vi "Process.vi"(8 "error in (no error)":errorcluster, 11 "SMO.UI":refnum<class "SMO.UI.lvclass">) -> (0 "error out":errorcluster, 3 "SMO.UI out":refnum<class "SMO.UI.lvclass">)   [LabVIEW 2013, in "SMO.UI.lvclass"]
uses:
  SMO.UI.lvclass
  SMO/Typedefs/Parent Call--Enum.ctl
  SMO/SMO.lvclass
panel:
  in  "OK":bool
  out "Copyright":string="JKI State Machine Objects™\nhttp://jki.net/state-machine-objects/\nCopyright (C) 2005-2015, JKI <info@jki.net>\nALL RIGHTS RESERVED\n\nFor instructions on how to use the JKI State Machine Objects, examples and video tutorials, visit:\nhttp://jki.net/state-machine-objects/\n"
  # "JKI SMO UI"
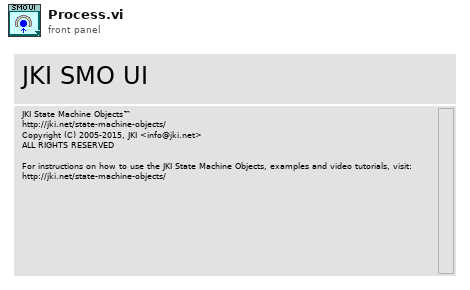
[diagram p1: front panel]
types:
  T1 = typedef "SMO.lvclass/Parent Call--Enum.ctl" = enum16{"Allows parent to run", "Does not request parent to run"}
  T2 = enum32{"invalid app kind", "Development System", "Run Time System", "Student Edition", "Embedded LabVIEW", "Evaluation", "Custom"}
  T3 = enum32{"Invalid", "Standard", "Closed", "Hidden", "Minimized", "Maximized"}
  T4 = cluster{"Core":cluster{"Current VI Reference":refnum<vi>, "Close Panel on Exit?":bool, "error":errorcluster}, "Self Ref":refnum<class "SMO.UI.lvclass">}
  T5 = cluster{"Current VI Reference":refnum<vi>, "Close Panel on Exit?":bool, "error":errorcluster}
  T6 = typedef "SMO.lvclass/Protected Events.ctl" = cluster{"StopProcesses":refnum<user-event>, "AbortProcesses":refnum<user-event>}
  T7 = typedef "SMO.UI.lvclass/PrivateEvents--Cluster.ctl" = cluster{"Show-Hide UI":refnum<user-event>}
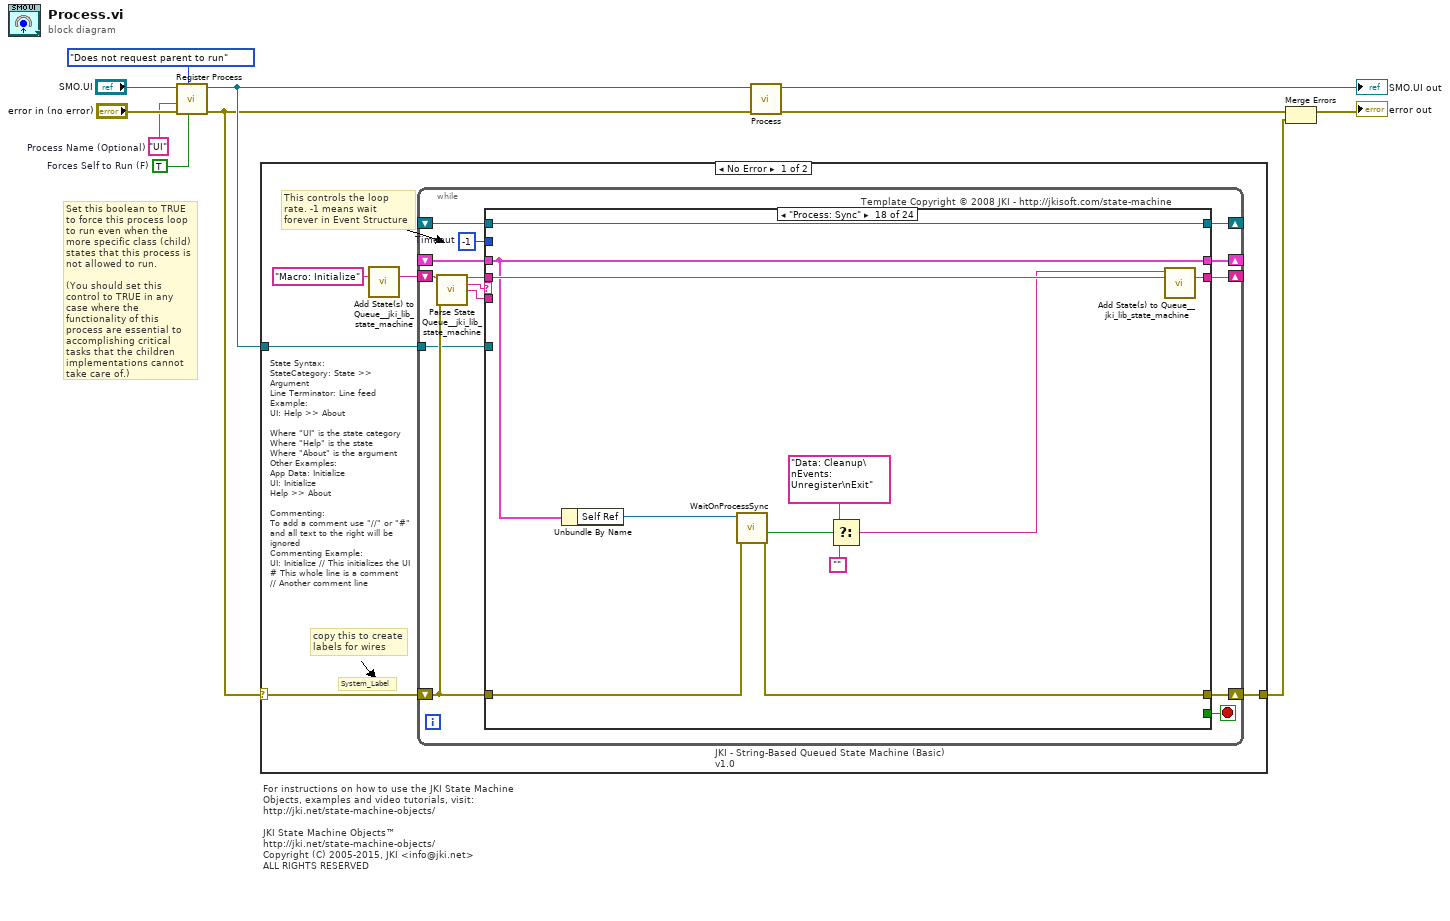
[diagram p0: block diagram]
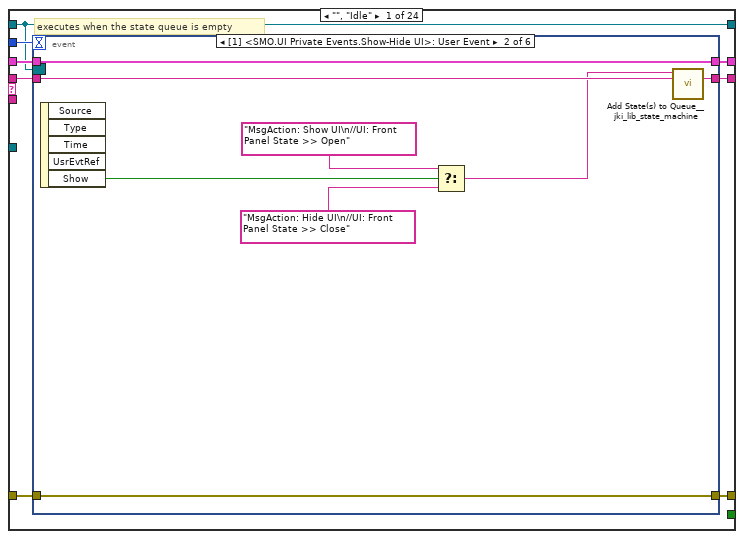
[diagram p2: hidden frame]
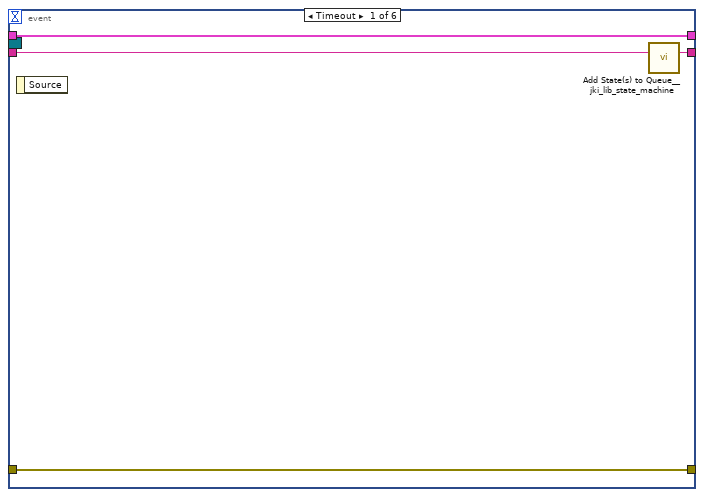
[diagram p3: hidden frame]
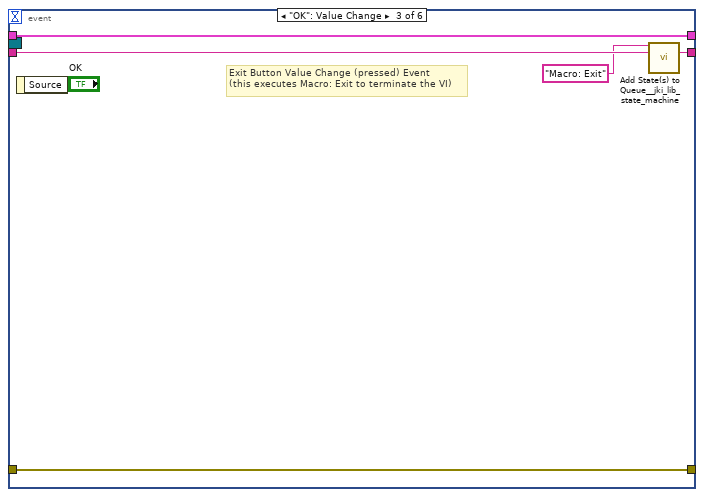
[diagram p4: hidden frame]
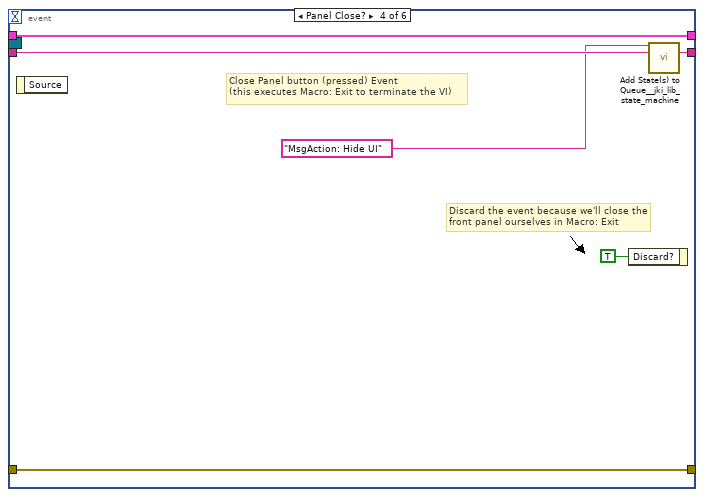
[diagram p5: hidden frame]
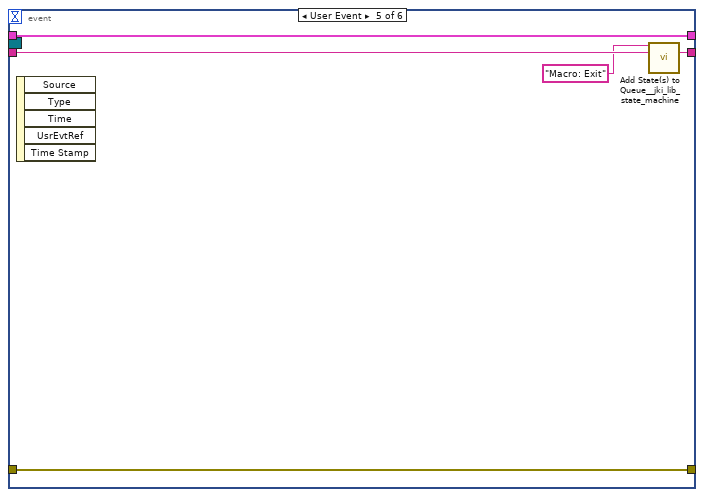
[diagram p6: hidden frame]
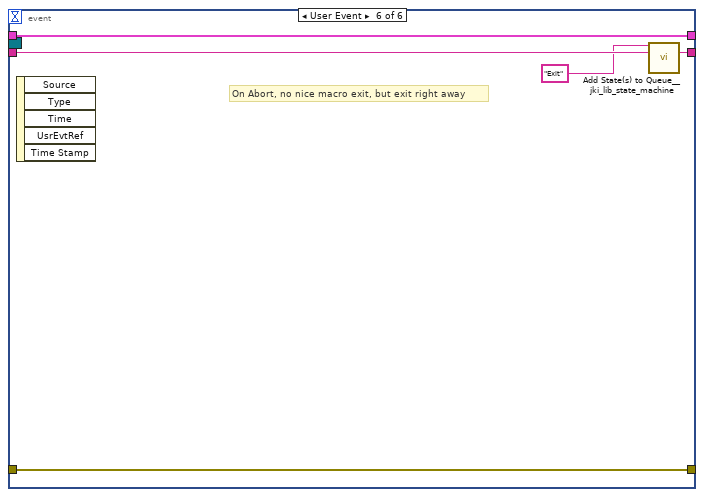
[diagram p7: hidden frame]
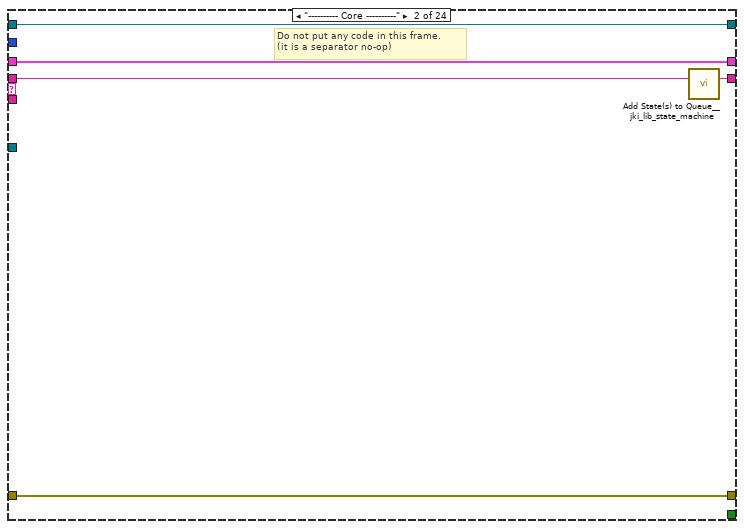
[diagram p8: hidden frame]
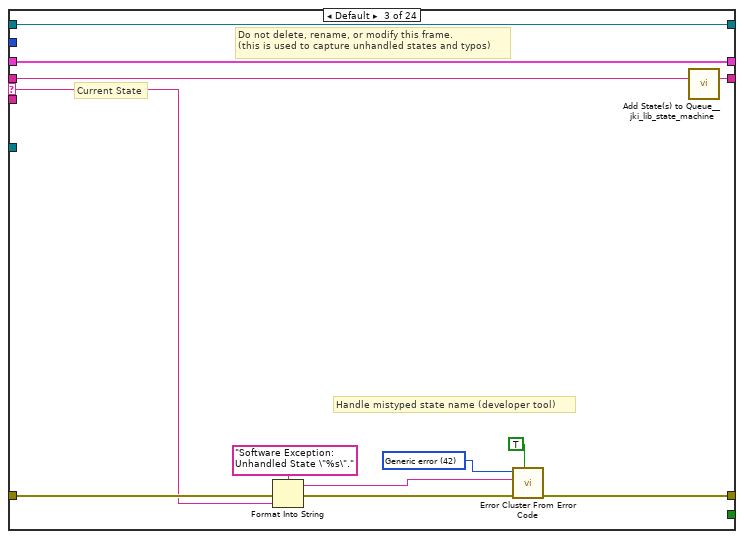
[diagram p9: hidden frame]
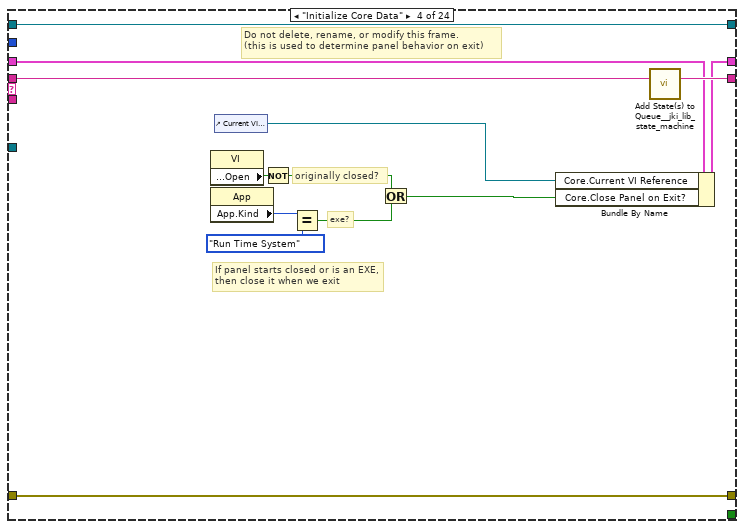
[diagram p10: hidden frame]
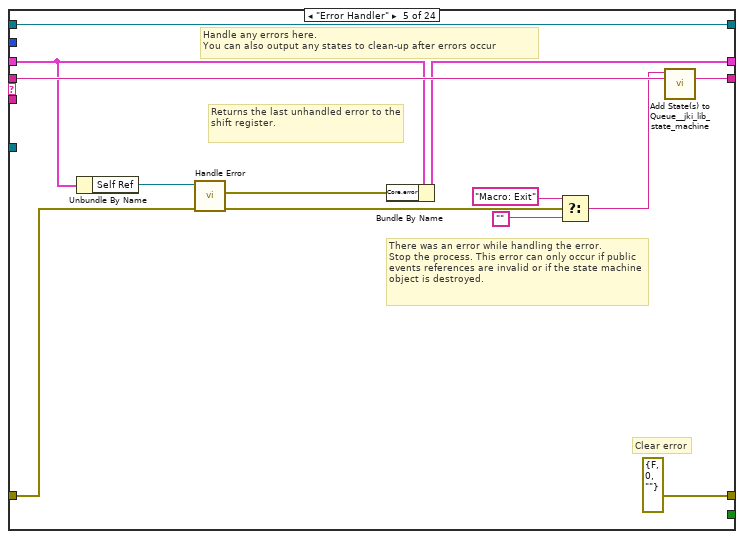
[diagram p11: hidden frame]
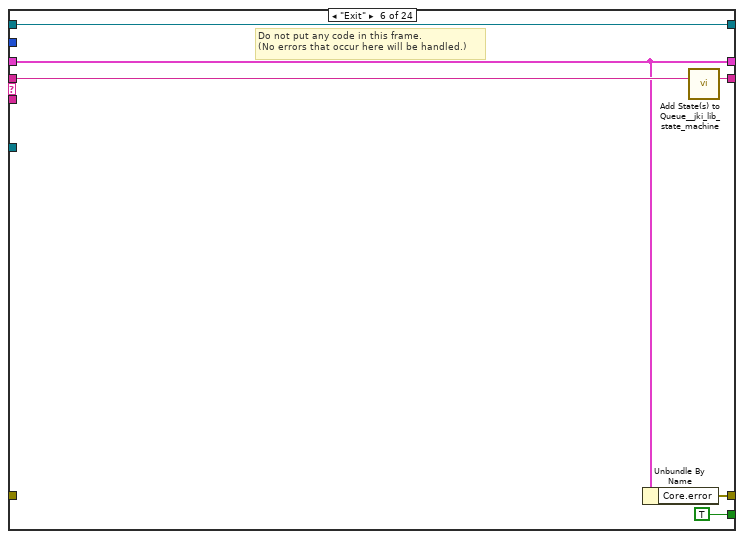
[diagram p12: hidden frame]
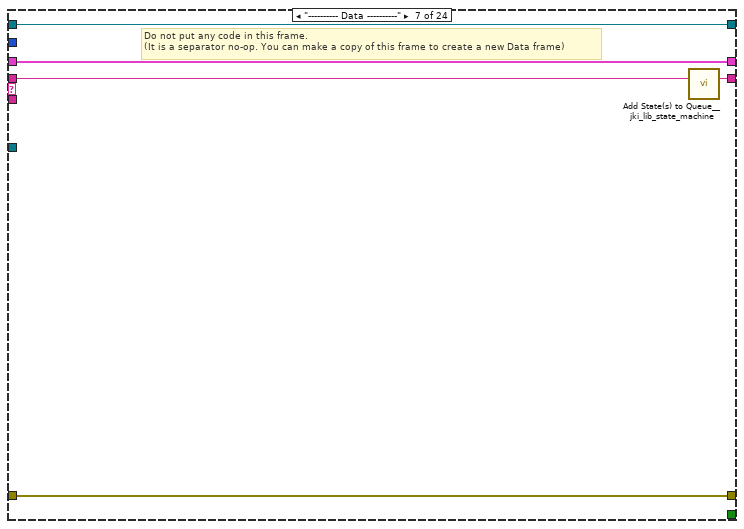
[diagram p13: hidden frame]
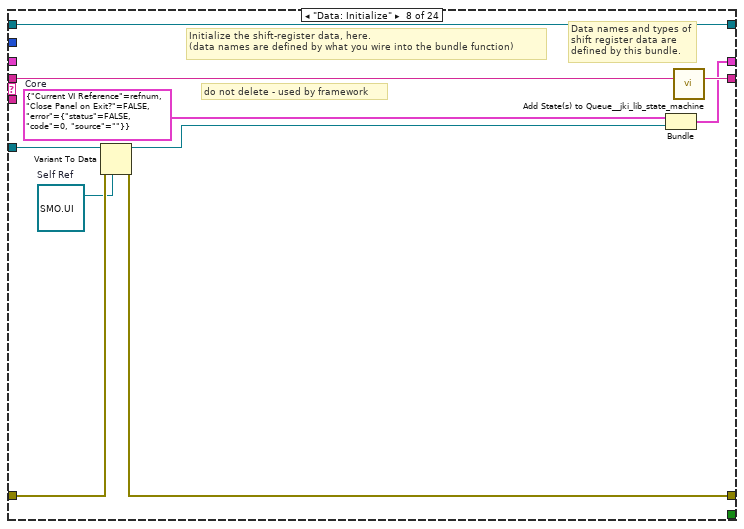
[diagram p14: hidden frame]
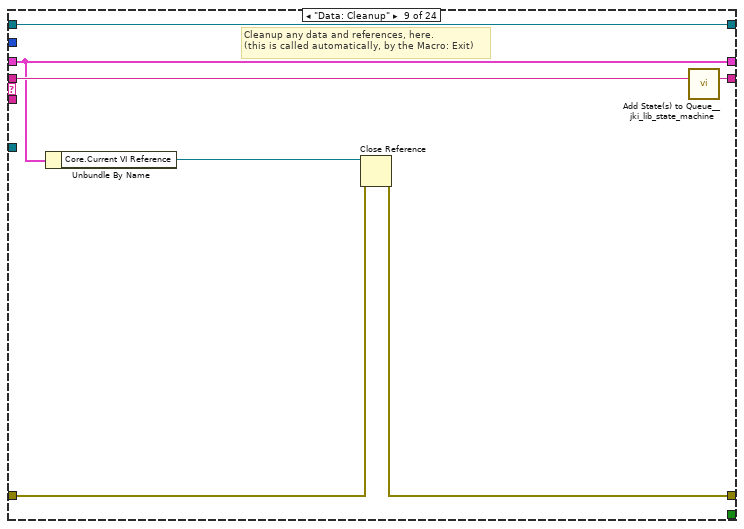
[diagram p15: hidden frame]
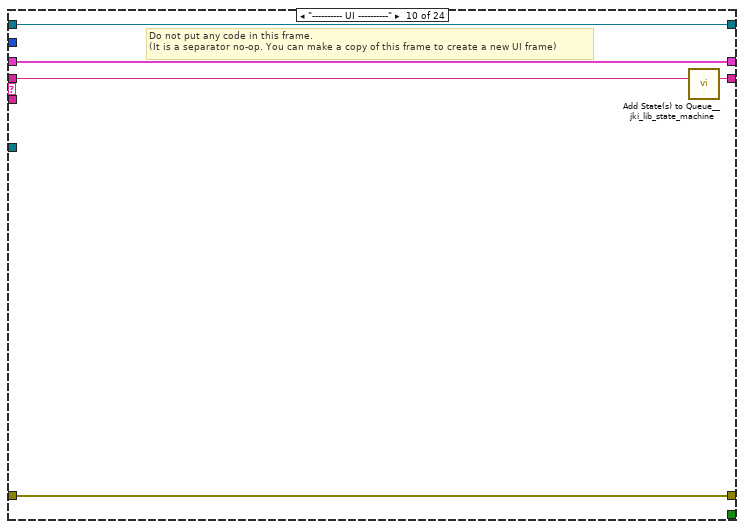
[diagram p16: hidden frame]
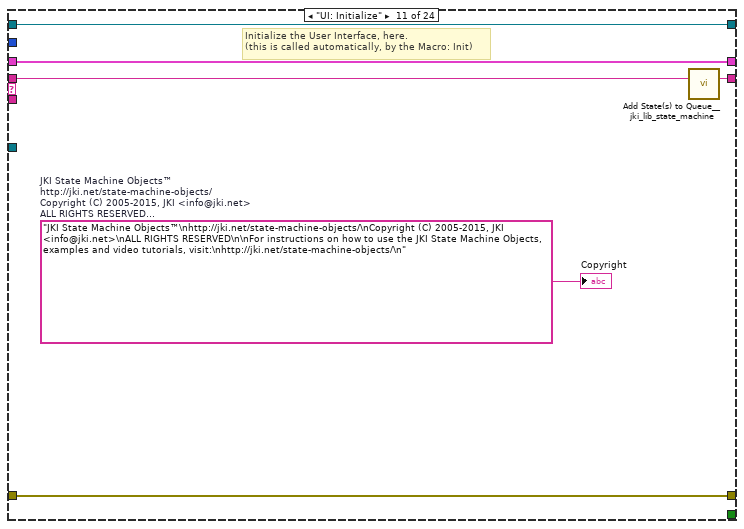
[diagram p17: hidden frame]
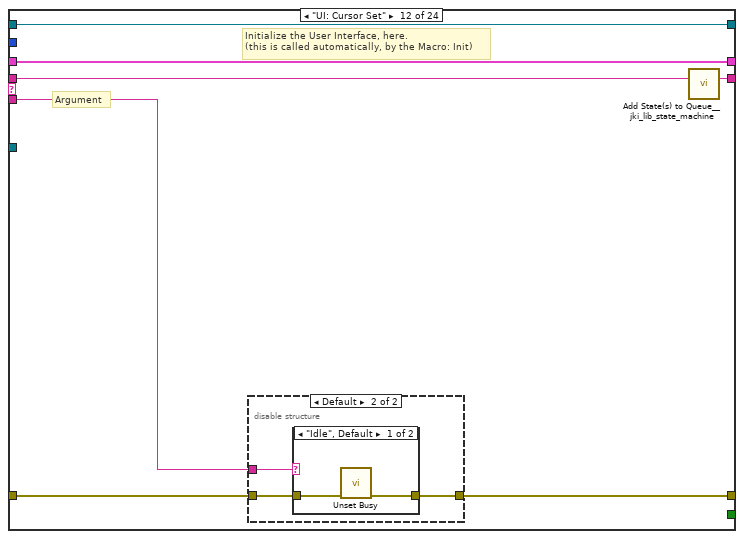
[diagram p18: hidden frame]
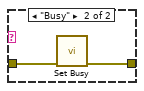
[diagram p20: hidden frame]
diagram:
  w2 = TRUE  # Forces Self to Run (F)
  w4 = "UI"  # Process Name (Optional)
  # "Set this boolean to TRUE to force this process loop to run even when the more specific class (child) states that this process is not allowed to run.\n\n(You should set this control to TRUE in any case where the functionality of this process are essential to accomplishing critical tasks that the children implementations cannot take care of.)"
  # "For instructions on how to use the JKI State Machine Objects, examples and video tutorials, visit:\nhttp://jki.net/state-machine-objects/\n\nJKI State Machine Objects™\nhttp://jki.net/state-machine-objects/\nCopyright (C) 2005-2015, JKI <info@jki.net>\nALL RIGHTS RESERVED"
  n1 = call "Register Process.vi"("Forces Self to Run (F)"=w2, "Parent Call"=Parent_Call--Enum."Does not request parent to run", "error in (no error)"="error in (no error)", "Process Name (optional)"=w4, "SMO"="SMO.UI") -> ("error out"=w10:errorcluster, "SMO out"=w11:refnum<class "SMO.UI.lvclass">)  [unwired: 5 in]
  n2 = case shown="No Error" w10 {
    selector: w10 -> [w13 w298]
    tunnel: w11 -> [w14 _]
    tunnel: [w12 w298] -> w8
    frame No Error {
      # "State Syntax:\nStateCategory: State >> Argument\nLine Terminator: Line feed\nExample:\nUI: Help >> About\n\nWhere \"UI\" is the state category\nWhere \"Help\" is the state\nWhere \"About\" is the argument\nOther Examples:\nApp Data: Initialize\nUI: Initialize\nHelp >> About\n\nCommenting:\nTo add a comment use \"//\" or \"#\" and all text to the right will be ignored\nCommenting Example:\nUI: Initialize // This initializes the UI\n# This whole line is a comment\n// Another comment line"
      # "copy this to create labels for wires"
      # "This controls the loop rate. -1 means wait forever in Event Structure"
      # "System_Label"
      n3 = call <vilib>:"Add State(s) to Queue__jki_lib_state_machine.vi"("State(s) in (\"\")"="Macro: Initialize") -> ("States Out"=w16:string)  [unwired: 14 in]
      n4 = while "JKI - String-Based Queued State Machine (Basic) v1.0" {
        shift-right: [w23] -> _
        shift-left: _ -> [w22]
        shift-right: [w26] -> w12
        shift-left: w13 -> [w20]
        shift-right: [w25] -> _
        shift-left: w16 -> [w27]
        tunnel: w14 -> [w19]
        shift-right: [w18] -> _
        shift-left: _ -> [w17]
        stop <- w24 stop-if-true
        w21 = -1  # Timeout
        # "Template Copyright © 2008 JKI - http://jkisoft.com/state-machine"
        n5 = call <vilib>:"Parse State Queue__jki_lib_state_machine.vi"("State Queue"=w27, "Error In (no error)"=w20) -> ("Remaining States"=w29:string, "Current State"=w30:string, "Arguments"=w28:string)  [unwired: 11 in]
        n6 = case shown="\"Process: Sync\"" w30 {
          selector: w30 -> [_ _ w78 _ _ _ _ _ _ _ _ _ _ _ _ _ _ _ _ _ _ _ _ _]
          tunnel: w29 -> [w38 w76 w82 w101 w114 w120 w125 w135 w142 w147 w153 w160 w176 w208 w217 w231 w236 w247 w252 w264 w270 w275 w283 w293]
          tunnel: w28 -> [_ _ _ _ _ _ _ _ _ _ _ w154 w172 _ _ _ _ _ _ _ _ _ _ _]
          tunnel: w22 -> [w36 w73 w80 w92 w110 w115 w122 _ w137 w144 w151 w158 w174 w205 w213 w222 w233 w244 w249 w262 w268 w272 w280 w290]
          tunnel: [w35 w74 w84 w98 errorcluster {"status"=FALSE, "code"=0, "source"=""} ("error out") w116 w123 w127 w138 w145 w150 w155 w169 w206 w215 w229 w234 w238 w250 w260 w266 w273 w277 w284] -> w26
          tunnel: w20 -> [w34 w74 w83 w98 w107 _ w123 w132 w139 w145 w150 w156 w170 w206 w215 w229 w234 w239 w250 w253 w266 w273 w278 w288]
          tunnel: [w37 w75 w81 w100 w113 w119 w124 w134 w141 w146 w152 w159 w175 w207 w216 w230 w235 w246 w251 w263 w269 w274 w282 w292] -> w25
          tunnel: [_ _ _ _ _ TRUE _ _ _ _ _ _ _ _ _ _ _ _ _ _ _ _ _ _] -> w24
          tunnel: [w33 w73 w80 w99 w109 w115 w122 w133 w137 w144 w151 w158 w174 w205 w213 w222 w233 w244 w249 w262 w268 w272 w280 w290] -> w23
          tunnel: w21 -> [w32 _ _ _ _ _ _ _ _ _ _ _ _ _ _ _ _ _ _ _ _ _ _ _]
          tunnel: w19 -> [_ _ _ _ _ _ _ w131 _ _ _ _ _ _ _ _ _ _ _ _ _ _ _ _]
          tunnel: [w31 w72 w77 w89 w112 w117 w121 w130 w136 w143 w149 w157 w173 w204 w214 w223 w232 w245 w248 w259 w267 w271 w281 w291] -> w18
          tunnel: w17 -> [w31 w72 w77 w89 w112 w117 w121 w130 w136 w143 w149 w157 w173 w204 w214 w223 w232 w245 w248 _ w267 w271 w281 w291]
          frame "", "Idle" {
            # "executes when the state queue is empty"
            n7 = event shown="[1] <SMO.UI Private Events.Show-Hide UI>: User Event" {
              selector: w31 -> [_ _ _ _ _ _]
              dyn-events: _ -> [_ _ _ _ _ _]
              timeout: w32 -> [_ _ _ _ _ _]
              tunnel: w38 -> [w42 w50 w55 w61 w66 w71]
              tunnel: [w41 w49 w54 w60 w65 w70] -> w37
              tunnel: w36 -> [w39 w47 w52 w57 w63 w68]
              tunnel: [w40 w48 w53 w59 w64 w69] -> w35
              tunnel: w34 -> [w40 w48 w53 w59 w64 w69]
              tunnel: [w39 w47 w52 w57 w63 w68] -> w33
              event Timeout {
                n8 = event-data() -> ()  [unwired: 1 in, 1 out]
                n9 = call <vilib>:"Add State(s) to Queue__jki_lib_state_machine.vi"("State(s) in (\"\")"=w42) -> ("States Out"=w41:string)  [unwired: 14 in]
              }
              event User Event {
                n10 = event-data() -> ("Show"=w46:bool)  [unwired: 1 in, 4 out]
                n11 = Select(t="MsgAction: Show UI\n//UI: Front Panel State >> Open" ("State(s) in Front (\"\")"), s=w46, f="MsgAction: Hide UI\n//UI: Front Panel State >> Close" ("State(s) in Front (\"\")")) -> (s? t:f=w43:string)
                n12 = call <vilib>:"Add State(s) to Queue__jki_lib_state_machine.vi"("State(s) in Front (\"\")"=w43, "State(s) in (\"\")"=w50) -> ("States Out"=w49:string)  [unwired: 13 in]
              }
              event "OK": Value Change {
                # "Exit Button Value Change (pressed) Event\n(this executes Macro: Exit to terminate the VI)"
                n13 = event-data() -> ()  [unwired: 1 in, 1 out]
                n14 = call <vilib>:"Add State(s) to Queue__jki_lib_state_machine.vi"("State(s) in Front (\"\")"="Macro: Exit", "State(s) in (\"\")"=w55) -> ("States Out"=w54:string)  [unwired: 13 in]
              }
              event Panel Close? {
                # "Discard the event because we'll close the front panel ourselves in Macro: Exit"
                # "Close Panel button (pressed) Event\n(this executes Macro: Exit to terminate the VI)"
                n15 = event-data() -> ()  [unwired: 1 in, 1 out]
                n16 = event-data("Discard?"=TRUE) -> ()  [unwired: 1 in, 1 out]
                n17 = call <vilib>:"Add State(s) to Queue__jki_lib_state_machine.vi"("State(s) in Front (\"\")"="MsgAction: Hide UI", "State(s) in (\"\")"=w61) -> ("States Out"=w60:string)  [unwired: 13 in]
              }
              event User Event {
                n18 = event-data() -> ()  [unwired: 1 in, 5 out]
                n19 = call <vilib>:"Add State(s) to Queue__jki_lib_state_machine.vi"("State(s) in Front (\"\")"="Macro: Exit", "State(s) in (\"\")"=w66) -> ("States Out"=w65:string)  [unwired: 13 in]
              }
              event User Event {
                # "On Abort, no nice macro exit, but exit right away"
                n20 = event-data() -> ()  [unwired: 1 in, 5 out]
                n21 = call <vilib>:"Add State(s) to Queue__jki_lib_state_machine.vi"("State(s) in Front (\"\")"="Exit", "State(s) in (\"\")"=w71) -> ("States Out"=w70:string)  [unwired: 13 in]
              }
            }
          }
          frame "---------- Core ----------" {
            # "Do not put any code in this frame.\n(it is a separator no-op)"
            n22 = call <vilib>:"Add State(s) to Queue__jki_lib_state_machine.vi"("State(s) in (\"\")"=w76) -> ("States Out"=w75:string)  [unwired: 14 in]
          }
          frame Default {
            w87 = 42 items=["No error", "Argument error", "Memory is full", "Out of zone", "End of file", "File already open", "Generic file I/O error", "File not found", "File permission error", "Disk is full", "Duplicate path", "Too many files open", "System feature not enabled", "Resource file not found", "Cannot add resource", "Resource not found", "Image not found", "Image memory error", "Pen does not exist", "Config type invalid", "Config token not found", "Config parse error", "Config memory error", "Bad external code format", "Bad external code offset", "External code not present", "Null window", "Destroy window error", "Null menu", "Print aborted", "Bad print record", "Print driver error", "Windows error during printing", "Memory error during printing", "Print dialog error", "Generic print error", "Invalid device refnum", "Device not found", "Device parameter error", "Device unit error", "Cannot open device", "Device call aborted", "Generic error", "Cancelled by user", "Object ID too low", "Object ID too high", "Object not in heap", "Unknown heap", "Unknown object (invalid DefProc)", "Unknown object (DefProc not in table)", "Message out of range", "Invalid (null) method", "Unknown message", "Manager call not supported", "Bad address", "Network operation in progress", "Network operation timed out", "Connection is busy", "Network attribute not supported", "Network error", "Address in use", "System out of memory", "Connection aborted", "Connection refused", "Not connected", "Already connected", "Connection closed", "Initialization error (interapplication manager)", "Bad occurrence", "Wait on unbound occurrence handler", "Occurrence queue overflow", "Datalog type conflict", "Unused", "Unrecognized type (interapplication manager)", "Memory corrupt", "Failed to make temporary DLL", "Old CIN version", "Drag socket not found", "Failed to load drop-object", "Failed to register OLE object", "Failed to release OLE object", "Format specifier type mismatch", "Unknown format specifier", "Too few format specifiers", "Too many format specifiers", "Scan failed", "Newer CIN version", "Error converting to variant", "Runtime menu error", "Password tampered", "Variant attribute not found", "Incompatible variant data type", "Event data is not available", "Event Store is not present", "Occurrence is not found", "Event Queue is not created", "Event info is not available", "Refnum passed is NULL", "Error retrieving Class GUID", "Error retrieving CoClass GUID", "Error retrieving TypeLib GUID.", "Bad built application magic bytes.", "Specific driver is different from the specific driver associated with the Logical Name.", "There is no session opened to the class driver.", "Max Error", "MAX - Error with config objects", "MAX - Error loading configuration", "MAX - Group not supported"]
            # "Current State"
            # "Do not delete, rename, or modify this frame.\n(this is used to capture unhandled states and typos)"
            # "Handle mistyped state name (developer tool)"
            n23 = Format Into String(format string="Software Exception: Unhandled State \"%s\"." ("message"), error in=w83, w78) -> (resulting string=w86:string, error out=w85:errorcluster)  [unwired: 1 in]
            n24 = call <vilib>:"Error Cluster From Error Code.vi"("show call chain? (False)"=TRUE, "error in (no error)"=w85, "error message (\"\")"=w86, "error code (0)"=w87) -> ("error out"=w84:errorcluster)  [unwired: 5 in]
            n25 = call <vilib>:"Add State(s) to Queue__jki_lib_state_machine.vi"("State(s) in (\"\")"=w82) -> ("States Out"=w81:string)  [unwired: 14 in]
          }
          frame "Initialize Core Data" {
            # "Do not delete, rename, or modify this frame.\n(this is used to determine panel behavior on exit)"
            # "originally closed?"
            # "exe?"
            # "If panel starts closed or is an EXE, then close it when we exit"
            n26 = property class="VI"() -> ("Front Panel.Open"=w97:bool)  [unwired: 2 in, 2 out]
            n27 = property class="App"() -> ("App.Kind"=w96:T2)  [unwired: 2 in, 2 out]
            n28 = control-ref of="Current VI Reference"() -> (w90:refnum<vi>)
            n29 = Not(x=w97) -> (.not. x?=w94:bool)
            n30 = Equal?(x=w96, y=T2."Run Time System" ("Application:Kind")) -> (x = y?=w93:bool)
            n31 = Or(x=w94, y=w93) -> (x .or. y?=w91:bool)
            n32 = Bundle By Name(cluster=w92, "Core.Current VI Reference"=w90, "Core.Close Panel on Exit?"=w91) -> (w99:T4)
            n33 = call <vilib>:"Add State(s) to Queue__jki_lib_state_machine.vi"("State(s) in (\"\")"=w101) -> ("States Out"=w100:string)  [unwired: 14 in]
          }
          frame "Error Handler" {
            # "Returns the last unhandled error to the shift register."
            # "There was an error while handling the error.\nStop the process. This error can only occur if public events references are invalid or if the state machine object is destroyed."
            # "Handle any errors here.\nYou can also output any states to clean-up after errors occur"
            # "Clear error"
            n34 = Unbundle By Name(w110) -> ("Self Ref"=w111:refnum<class "SMO.UI.lvclass">)
            n35 = call-dynamic "Handle Error.vi"("error in"=w107, "SMO"=w111) -> ("handling error"=w105:errorcluster, "Unhandled error"=w108:errorcluster)  [unwired: 7 in, 1 out]
            n36 = Bundle By Name(cluster=w110, "Core.error"=w108) -> (w109:T4)
            n37 = Select(t="Macro: Exit", s=w105, f="") -> (s? t:f=w102:string)
            n38 = call <vilib>:"Add State(s) to Queue__jki_lib_state_machine.vi"("State(s) in Front (\"\")"=w102, "State(s) in (\"\")"=w114) -> ("States Out"=w113:string)  [unwired: 13 in]
          }
          frame "Exit" {
            # "Do not put any code in this frame.\n(No errors that occur here will be handled.)"
            n39 = Unbundle By Name(w115) -> ("Core.error"=w116:errorcluster)
            n40 = call <vilib>:"Add State(s) to Queue__jki_lib_state_machine.vi"("State(s) in (\"\")"=w120) -> ("States Out"=w119:string)  [unwired: 14 in]
          }
          frame "---------- Data ----------" {
            # "Do not put any code in this frame.\n(It is a separator no-op. You can make a copy of this frame to create a new Data frame)"
            n41 = call <vilib>:"Add State(s) to Queue__jki_lib_state_machine.vi"("State(s) in (\"\")"=w125) -> ("States Out"=w124:string)  [unwired: 14 in]
          }
          frame "Data: Initialize" {
            w126 = T5 {"Current VI Reference"=refnum, "Close Panel on Exit?"=FALSE, "error"={"status"=FALSE, "code"=0, "source"=""}}  # Core
            w129 = refnum<class "SMO.UI.lvclass"> refnum  # Self Ref
            # "do not delete - used by framework"
            # "Data names and types of shift register data are defined by this bundle."
            # "Initialize the shift-register data, here.\n(data names are defined by what you wire into the bundle function)"
            n42 = Variant To Data(error in=w132, type=w129, Variant=w131) -> (data=w128:refnum<class "SMO.UI.lvclass">, error out=w127:errorcluster)
            n43 = Bundle("Core"=w126, "Self Ref"=w128) -> (w133:T4)  [unwired: 1 in]
            n44 = call <vilib>:"Add State(s) to Queue__jki_lib_state_machine.vi"("State(s) in (\"\")"=w135) -> ("States Out"=w134:string)  [unwired: 14 in]
          }
          frame "Data: Cleanup" {
            # "Cleanup any data and references, here.\n(this is called automatically, by the Macro: Exit)"
            n45 = Unbundle By Name(w137) -> ("Core.Current VI Reference"=w140:refnum<vi>)
            n46 = Close Reference(reference=w140, error in (no error)=w139) -> (error out=w138:errorcluster)
            n47 = call <vilib>:"Add State(s) to Queue__jki_lib_state_machine.vi"("State(s) in (\"\")"=w142) -> ("States Out"=w141:string)  [unwired: 14 in]
          }
          frame "---------- UI ----------" {
            # "Do not put any code in this frame.\n(It is a separator no-op. You can make a copy of this frame to create a new UI frame)"
            n48 = call <vilib>:"Add State(s) to Queue__jki_lib_state_machine.vi"("State(s) in (\"\")"=w147) -> ("States Out"=w146:string)  [unwired: 14 in]
          }
          frame "UI: Initialize" {
            w148 = "JKI State Machine Objects™\nhttp://jki.net/state-machine-objects/\nCopyright (C) 2005-2015, JKI <info@jki.net>\nALL RIGHTS RESERVED\n\nFor instructions on how to use the JKI State Machine Objects, examples and video tutorials, visit:\nhttp://jki.net/state-machine-objects/\n"  # JKI State Machine Objects™ http://jki.net/state-machine-objects/ Copyright (C) 2005-2015, JKI <info@jki.net> ALL RIGHTS RESERVED  For instructions on how to use the JKI State Machine Objects, examples and video tutorials, visit: http://jki.net/state-machine-objects/
            # "Initialize the User Interface, here.\n(this is called automatically, by the Macro: Init)"
            n49 = call <vilib>:"Add State(s) to Queue__jki_lib_state_machine.vi"("State(s) in (\"\")"=w153) -> ("States Out"=w152:string)  [unwired: 14 in]
            "Copyright" <- w148
          }
          frame "UI: Cursor Set" {
            # "Argument"
            # "Initialize the User Interface, here.\n(this is called automatically, by the Macro: Init)"
            n50 = disable-structure shown="Default" {
              disable-tunnel: w156 -> [w161 w164]
              disable-tunnel: [w161 w163] -> w155
              disable-tunnel: w154 -> [_ w162]
              frame condition #0 {
              }
              frame condition #1 (active) {
                n51 = case shown="\"Idle\", Default" w162 {
                  tunnel: w164 -> [w166 w168]
                  tunnel: [w165 w167] -> w163
                  frame "Idle", Default {
                    n52 = call <vilib>:"Unset Busy.vi"("error in (no error)"=w166) -> ("error out"=w165:errorcluster)  [unwired: 10 in]
                  }
                  frame "Busy" {
                    n53 = call <vilib>:"Set Busy.vi"("error in (no error)"=w168) -> ("error out"=w167:errorcluster)  [unwired: 9 in, 1 out]
                  }
                }
              }
            }
            n54 = call <vilib>:"Add State(s) to Queue__jki_lib_state_machine.vi"("State(s) in (\"\")"=w160) -> ("States Out"=w159:string)  [unwired: 14 in]
          }
          frame "UI: Front Panel State" {
            # "Argument"
            # "Set Front Panel Open or Closed\n(Usage: \"UI: Front Panel State >> Open|Close\")"
            n55 = Unbundle By Name(w174) -> ("Core.Current VI Reference"=w171:refnum<vi>)
            n56 = disable-structure shown="Default" {
              disable-tunnel: w170 -> [w180 w203]
              disable-tunnel: [w179 w203] -> w169
              disable-tunnel: w171 -> [w178 _]
              disable-tunnel: w172 -> [w177 _]
              frame condition #0 (active) {
                n57 = case shown="\"Open\"" w177 {
                  tunnel: w180 -> [w184 w197]
                  tunnel: [w186 w198] -> w179
                  tunnel: w178 -> [w185 w195]
                  frame "Open" {
                    # "Open FP if not open or invalid"
                    n58 = property class="VI"(reference=w185, error in=w184) -> (reference out=w182:refnum<vi>, error out=w183:errorcluster, "FP.State"=w181:T3)
                    n59 = case shown="Default" w181 {
                      tunnel: [w189 w192] -> w186
                      tunnel: w183 -> [w188 w192]
                      tunnel: w182 -> [w187 _]
                      frame Default {
                        n60 = invoke class="VI" method="FP.Open"(reference=w187, error in=w188, "Activate"=TRUE, "State"=T3."Standard") -> (error out=w189:errorcluster)  [unwired: 1 in, 4 out]
                      }
                      frame "Invalid", "Standard" {
                      }
                    }
                  }
                  frame "Close", Default {
                    # "Close FP is not Closed or Invalid"
                    n61 = property class="VI"(reference=w195, error in=w197) -> (reference out=w194:refnum<vi>, error out=w196:errorcluster, "FP.State"=w193:T3)
                    n62 = case shown="Default" w193 {
                      tunnel: [w199 w202] -> w198
                      tunnel: w196 -> [w199 w201]
                      tunnel: w194 -> [_ w200]
                      frame "Invalid", "Closed" {
                      }
                      frame Default {
                        n63 = invoke class="VI" method="FP.Close"(reference=w200, error in=w201) -> (error out=w202:errorcluster)  [unwired: 1 in, 2 out]
                      }
                    }
                  }
                }
              }
              frame condition #1 {
              }
            }
            n64 = call <vilib>:"Add State(s) to Queue__jki_lib_state_machine.vi"("State(s) in (\"\")"=w176) -> ("States Out"=w175:string)  [unwired: 14 in]
          }
          frame "---------- Macro ----------" {
            # "Do not put any code in this frame.\n(It is a separator no-op. You can make a copy of this frame to create a new Macro frame)"
            n65 = call <vilib>:"Add State(s) to Queue__jki_lib_state_machine.vi"("State(s) in (\"\")"=w208) -> ("States Out"=w207:string)  [unwired: 14 in]
          }
          frame "Macro: Initialize" {
            w211 = "UI: Initialize\n//UI: Front Panel State >> Open"  # UI: Initialize //UI: Front Panel State >> Open
            # "Initialization Macro\n(This is called once, when the VI starts)"
            n66 = call <vilib>:"Add State(s) to Queue__jki_lib_state_machine.vi"("State(s) in Front (\"\")"="Data: Initialize\nInitialize Core Data\nEvents: Register", "State(s) in (\"\")"="Process: Sync", "State(s) at Back (\"\")"=w211) -> ("States Out"=w210:string)  [unwired: 12 in]
            n67 = call <vilib>:"Add State(s) to Queue__jki_lib_state_machine.vi"("State(s) in Front (\"\")"=w210, "State(s) in (\"\")"=w217) -> ("States Out"=w216:string)  [unwired: 13 in]
          }
          frame "Macro: Exit" {
            # "Exit Macro\n(This is called once, when the VI exits)"
            n68 = Unbundle By Name(w222) -> ("Core.Close Panel on Exit?"=w228:bool)
            n69 = Select(t="MsgAction: Hide UI", s=w228, f="") -> (s? t:f=w225:string)
            n70 = call <vilib>:"Add State(s) to Queue__jki_lib_state_machine.vi"("State(s) in Front (\"\")"="Data: Cleanup\nEvents: Unregister", "State(s) in (\"\")"="Process: Sync", "State(s) at Back (\"\")"="Exit") -> ("States Out"=w219:string)  [unwired: 12 in]
            n71 = call <vilib>:"Add State(s) to Queue__jki_lib_state_machine.vi"("State(s) in (\"\")"=w225, "State(s) at Back (\"\")"=w219) -> ("States Out"=w224:string)  [unwired: 13 in]
            n72 = call <vilib>:"Add State(s) to Queue__jki_lib_state_machine.vi"("State(s) in Front (\"\")"=w224, "State(s) in (\"\")"=w231) -> ("States Out"=w230:string)  [unwired: 13 in]
          }
          frame "---------- Process ----------" {
            # "Template Separator\n(You can make a copy of, or modify, this frame)"
            n73 = call <vilib>:"Add State(s) to Queue__jki_lib_state_machine.vi"("State(s) in (\"\")"=w236) -> ("States Out"=w235:string)  [unwired: 14 in]
          }
          frame "Process: Sync" {
            n74 = Unbundle By Name(w244) -> ("Self Ref"=w240:refnum<class "SMO.UI.lvclass">)
            n75 = call "WaitOnProcessSync.vi"("error in (no error)"=w239, "SMO"=w240) -> ("error out"=w238:errorcluster, "Don't run?"=w243:bool)  [unwired: 7 in, 1 out]
            n76 = Select(t="Data: Cleanup\nEvents: Unregister\nExit", s=w243, f="") -> (s? t:f=w237:string)
            n77 = call <vilib>:"Add State(s) to Queue__jki_lib_state_machine.vi"("State(s) in Front (\"\")"=w237, "State(s) in (\"\")"=w247) -> ("States Out"=w246:string)  [unwired: 13 in]
          }
          frame "---------- Events ----------" {
            # "Template Separator\n(You can make a copy of, or modify, this frame)"
            n78 = call <vilib>:"Add State(s) to Queue__jki_lib_state_machine.vi"("State(s) in (\"\")"=w252) -> ("States Out"=w251:string)  [unwired: 14 in]
          }
          frame "Events: Register" {
            n79 = Unbundle By Name(w262) -> ("Self Ref"=w258:refnum<class "SMO.UI.lvclass">)
            n80 = call "GetProtectedEvents.vi"("error in (no error)"=w253, "SMO"=w258) -> ("error out"=w254:errorcluster, "SMO Protected Events"=w261:T6, "SMO out"=w255:refnum<class "SMO.UI.lvclass">)  [unwired: 7 in]
            n81 = call "SMO.UI.GetPrivateEvents.vi"("error in (no error)"=w254, "SMO.UI"=w255) -> ("error out"=w256:errorcluster, "SMO.UI Private Events"=w257:T7)  [unwired: 7 in, 1 out]
            n82 = register-events(error in=w256, w261, w257) -> (reference out=w259:refnum<event-registration>, error out=w260:errorcluster)  [unwired: 1 in]
            n83 = call <vilib>:"Add State(s) to Queue__jki_lib_state_machine.vi"("State(s) in (\"\")"=w264) -> ("States Out"=w263:string)  [unwired: 14 in]
          }
          frame "Events: Unregister" {
            # "Your code here.\n(You can make a copy of, or modify, this frame)"
            n84 = Unregister For Events(event registration refnum=w267, error in=w266) -> (error out=w265:errorcluster)
            n85 = call <vilib>:"Clear Errors.vi"("error in (no error)"=w265) -> ()  [unwired: 6 in, 1 out]
            n86 = call <vilib>:"Add State(s) to Queue__jki_lib_state_machine.vi"("State(s) in (\"\")"=w270) -> ("States Out"=w269:string)  [unwired: 14 in]
          }
          frame "---------MsgAction---------" {
            # "MsgAction Separator\n(You can make a copy of, or modify, this frame)"
            n87 = call <vilib>:"Add State(s) to Queue__jki_lib_state_machine.vi"("State(s) in (\"\")"=w275) -> ("States Out"=w274:string)  [unwired: 14 in]
          }
          frame "MsgAction: Show UI" {
            n88 = Unbundle By Name(w280) -> ("Self Ref"=w279:refnum<class "SMO.UI.lvclass">)
            n89 = call-dynamic "Show User Interface.vi"("error in (no error)"=w278, "Show UI"=TRUE, "SMO.UI"=w279) -> ("error out"=w277:errorcluster)  [unwired: 7 in, 1 out]
            n90 = call <vilib>:"Add State(s) to Queue__jki_lib_state_machine.vi"("State(s) in (\"\")"=w283) -> ("States Out"=w282:string)  [unwired: 14 in]
          }
          frame "MsgAction: Hide UI" {
            n91 = Unbundle By Name(w290) -> ("Self Ref"=w289:refnum<class "SMO.UI.lvclass">)
            n92 = call-dynamic "Show User Interface.vi"("error in (no error)"=w288, "Show UI"=FALSE, "SMO.UI"=w289) -> ("error out"=w285:errorcluster, "SMO.UI out"=w286:refnum<class "SMO.UI.lvclass">)  [unwired: 7 in]
            n93 = case shown="No Error" w285 {
              selector: w285 -> [w295 w297]
              tunnel: w286 -> [w296 _]
              tunnel: [w294 w297] -> w284
              frame No Error {
                n94 = call "NotifyUIHidden.vi"("error in (no error)"=w295, "SMO.UI"=w296) -> ("error out"=w294:errorcluster)  [unwired: 8 in, 1 out]
              }
              frame Error {
              }
            }
            n95 = call <vilib>:"Add State(s) to Queue__jki_lib_state_machine.vi"("State(s) in (\"\")"=w293) -> ("States Out"=w292:string)  [unwired: 14 in]
          }
        }
      }
    }
    frame Error {
    }
  }
  n96 = call-parent "Process.vi"("error in"=w10, "SMO"=w11) -> ("error out"=w9:errorcluster, "SMO out"=→"SMO.UI out":refnum<class "SMO.UI.lvclass">)  [unwired: 8 in]
  n97 = Merge Errors(w9, w8) -> (→"error out":errorcluster)
